vi "Get Topic Actor Look Up Table.vi"(8 "error in (no error)":errorcluster, 11 "Message Broker in":refnum<class "Message Broker.lvclass">) -> (0 "error out":errorcluster, 2 "Topic Actor Look Up Table":refnum<class "Topic Actor Look Up Table.lvclass">, 3 "Message Broker out":refnum<class "Message Broker.lvclass">)   [LabVIEW 2016, in "Stream Mediator.lvlib" / "Message Broker.lvclass"]
uses:
  <userlib>/Composed Systems/Stream/Mediator/Classes/Message Broker/Message Broker.lvclass
  <userlib>/Composed Systems/Stream/Mediator/Classes/Topic Actor Look Up Table/Topic Actor Look Up Table.lvclass
  <userlib>/Composed Systems/Stream/Mediator/Classes/Message Broker/Message Broker.lvclass/Message Broker.ctl
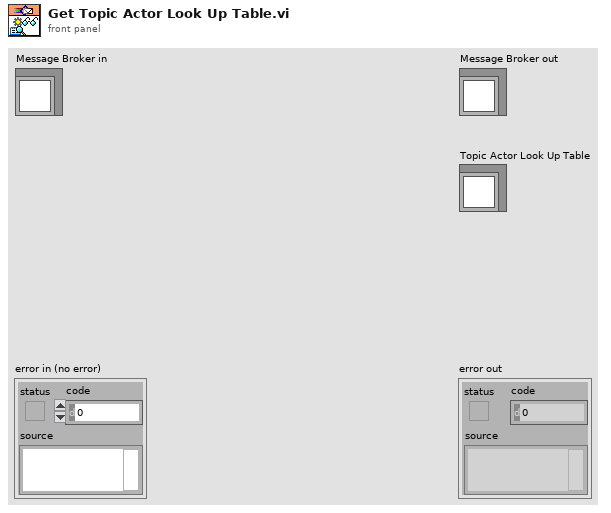
[diagram p1: front panel]
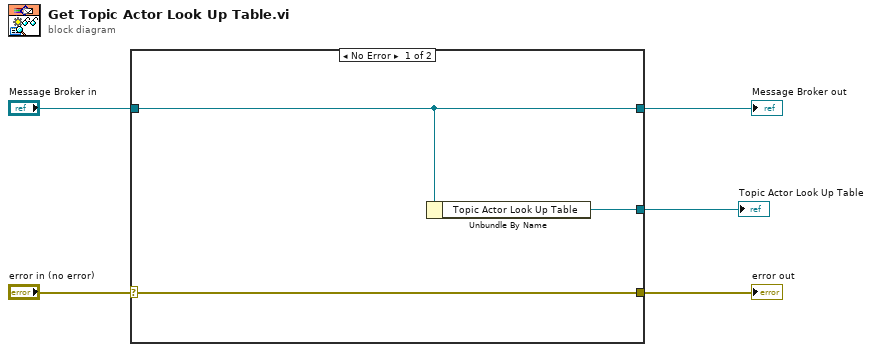
[diagram p0: block diagram]
diagram:
  n1 = case shown="No Error" "error in (no error)" {
    selector: "error in (no error)" -> [w8 w10]
    tunnel: [w8 w10] -> w4
    tunnel: [w7 w9] -> w2
    tunnel: "Message Broker in" -> [w7 w9]
    tunnel: [w6 _] -> w1
    frame No Error {
      n2 = Unbundle By Name(w7) -> ("Topic Actor Look Up Table"=w6:refnum<class "Topic Actor Look Up Table.lvclass">)
    }
    frame Error {
    }
  }
  "error out" <- w4
  "Message Broker out" <- w2
  "Topic Actor Look Up Table" <- w1
